vi "CAN Interface.vi"(8 "error in (no error)":errorcluster) -> (0 "error out":errorcluster, 2 "interface object out":refnum<k20>, 3 "Interface schließen?":bool)   [LabVIEW 2014]
uses:
  <vilib>/CANopenLib/CANOPEN.llb/CANopen BaudRate.ctl
  <vilib>/CANopenLib/CANOPEN.llb/CANopen Interface Create.vi
panel:
  in  "interface name":u32(ring) items=["CANopen01", "CANopen02", "CANopen03", "CANopen04", "CANopen05", "CANopen06", "CANopen07", "CANopen08", "CANopen09", "CANopen10", "CANopen11", "CANopen12", "CANopen13", "CANopen14", "CANopen15", "CANopen16", "CANopen17", "CANopen18", "CANopen19", "CANopen20", "CANopen21", "CANopen22", "CANopen23", "CANopen24", "CANopen25", "CANopen26", "CANopen27", "CANopen28", "CANopen29", "CANopen30", "CANopen31", "CANopen32"]
  in  "baud rate":T1 items=["1 Mbit/s"=0, "800 kbit/s"=1, "500 kbit/s"=2, "250 kbit/s"=3, "125 kbit/s"=4, "50 kbit/s"=6, "20 kbit/s"=7, "10 kbit/s"=8]
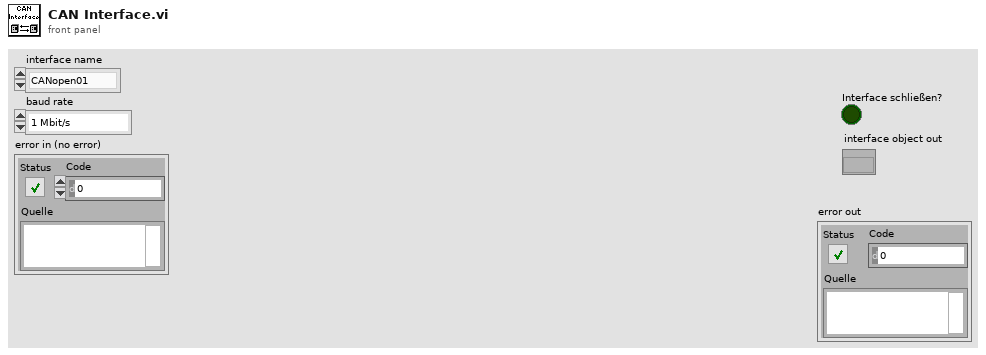
[diagram p1: front panel]
types:
  T1 = typedef "CANopen BaudRate.ctl" = u32
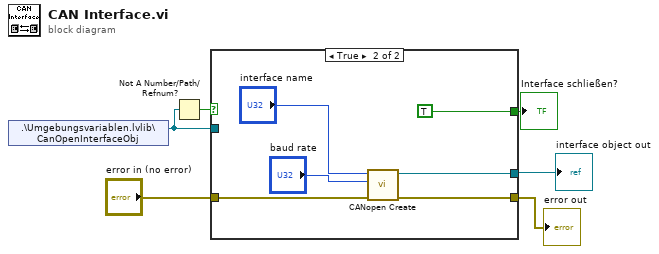
[diagram p0: block diagram]
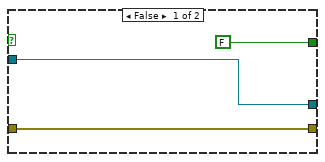
[diagram p2: hidden frame]
diagram:
  n1 = shared-variable ".\\Umgebungsvariablen.lvlib\\CanOpenInterfaceObj"() -> (w5:refnum<k20>)  [unwired: 1 in, 1 out]
  n2 = Not A Number/Path/Refnum?(number/path/refnum=w5) -> (NaN/Path/Refnum?=w6:bool)
  n3 = case shown="True" w6 {
    tunnel: [w8 w13] -> w3
    tunnel: "error in (no error)" -> [w8 w12]
    tunnel: [w9 w10] -> w1
    tunnel: w5 -> [w9 _]
    tunnel: [FALSE TRUE] -> w2
    frame False {
    }
    frame True {
      n4 = call-poly <vilib>:"CANopen Create.vi"("error in (no error)"=w12, "baud rate"="baud rate", "interface name"="interface name") -> ("error out"=w13:errorcluster, "interface object out"=w10:refnum<k20>)  [unwired: 7 in]
    }
  }
  "error out" <- w3
  "Interface schließen?" <- w2
  "interface object out" <- w1
